vi "InitAllowContinuousPressureAcquisition.vi"   [LabVIEW 2012]
uses:
  GlobalVariables/AllowContinuousPressureAcquisition.vi
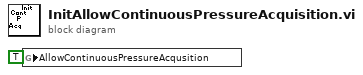
[diagram p0: block diagram]
diagram:
  n1 = global write "AllowContinuousPressureAcquisition.vi" "AllowContinuousPressureAcqusition"(TRUE) -> ()
